vi "Write Data To File.vi"(9 "Default Path":path, 10 "Path":path, 11 "Measurements":string[][](array[string])) -> ()   [LabVIEW 2018]
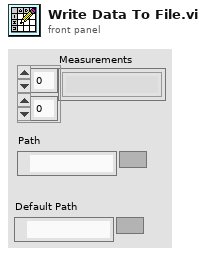
[diagram p1: front panel]
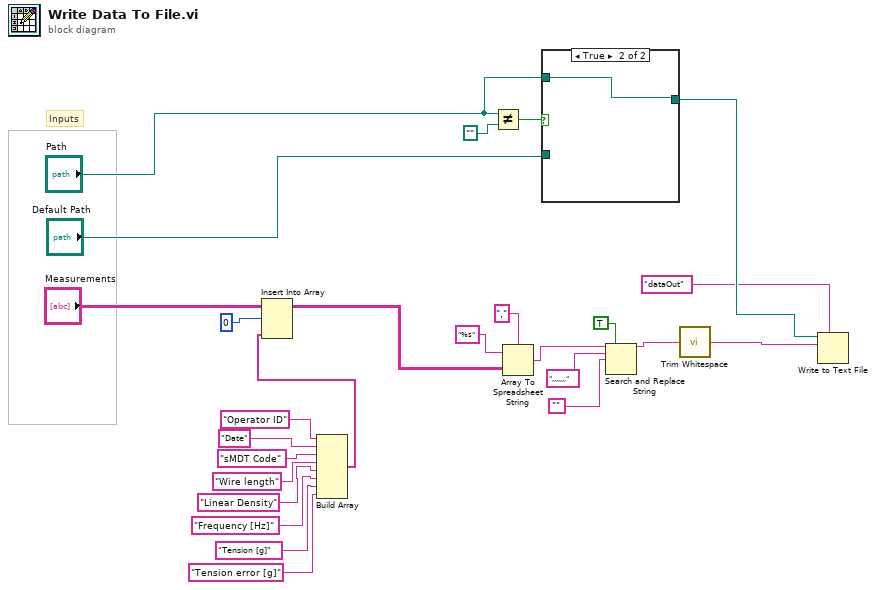
[diagram p0: block diagram]
diagram:
  # "Inputs"
  n1 = Build Array("Operator ID", "Date", "sMDT Code", "Wire length", "Linear Density", "Frequency [Hz]", "Tension [g]", "Tension error [g]") -> (w20:string[])
  n2 = Insert Into Array(array="Measurements", index (row)=0, new element=w20) -> (w21:string[][])  [unwired: 1 in]
  n3 = Not Equal?(x="Path", y=path "") -> (x != y?=w23:bool)
  n4 = Array To Spreadsheet String(delimiter (Tab)=",", array=w21, 3:"%s") -> (spreadsheet string=w13:string)
  n5 = case shown="True" w23 {
    tunnel: [w27 w28] -> w26
    tunnel: "Path" -> [_ w28]
    tunnel: "Default Path" -> [w27 _]
    frame False {
    }
    frame True {
    }
  }
  n6 = Search and Replace String(replace all?=TRUE, input string=w13, search string=",,,,,,,", replace string="") -> (result string=w17:string)  [unwired: 4 in, 3 out]
  n7 = call <vilib>:"Trim Whitespace.vi"("string"=w17) -> ("trimmed string"=w18:string)  [unwired: 1 in]
  n8 = Write to Text File(prompt (Choose or enter file path)="dataOut", file (use dialog)=w26, text=w18) -> ()  [unwired: 1 in, 3 out]
